vi "crossover detection.vi"(7 "reference line":dbl format="%#_13g", 8 "error in":errorcluster, 9 "Plot":dbl[][](array[numeric])) -> (0 "error out":errorcluster, 2 "crossovers":dbl[](array[numeric]))   [LabVIEW 2014]
panel:
  out "debouncing negative e":i32
  out "debouncing positive e.":i32
  out "n.e.c. validated":dbl[](array[numeric])
  out "p.e.c. validated":dbl[](array[numeric])
  out "positive edge\ncrossovers (x value)":dbl[](array[numeric])
  out "negative edge\ncorssovers (x value)":dbl[](array[numeric])
  # "For testing only"
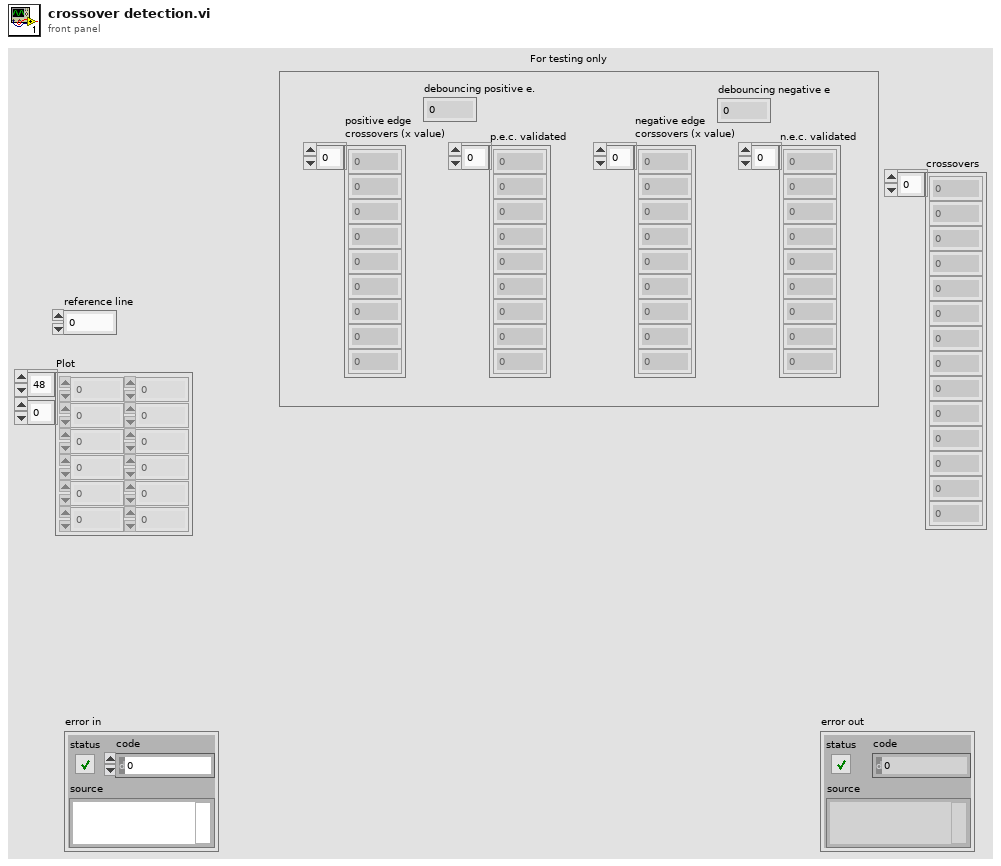
[diagram p1: front panel]
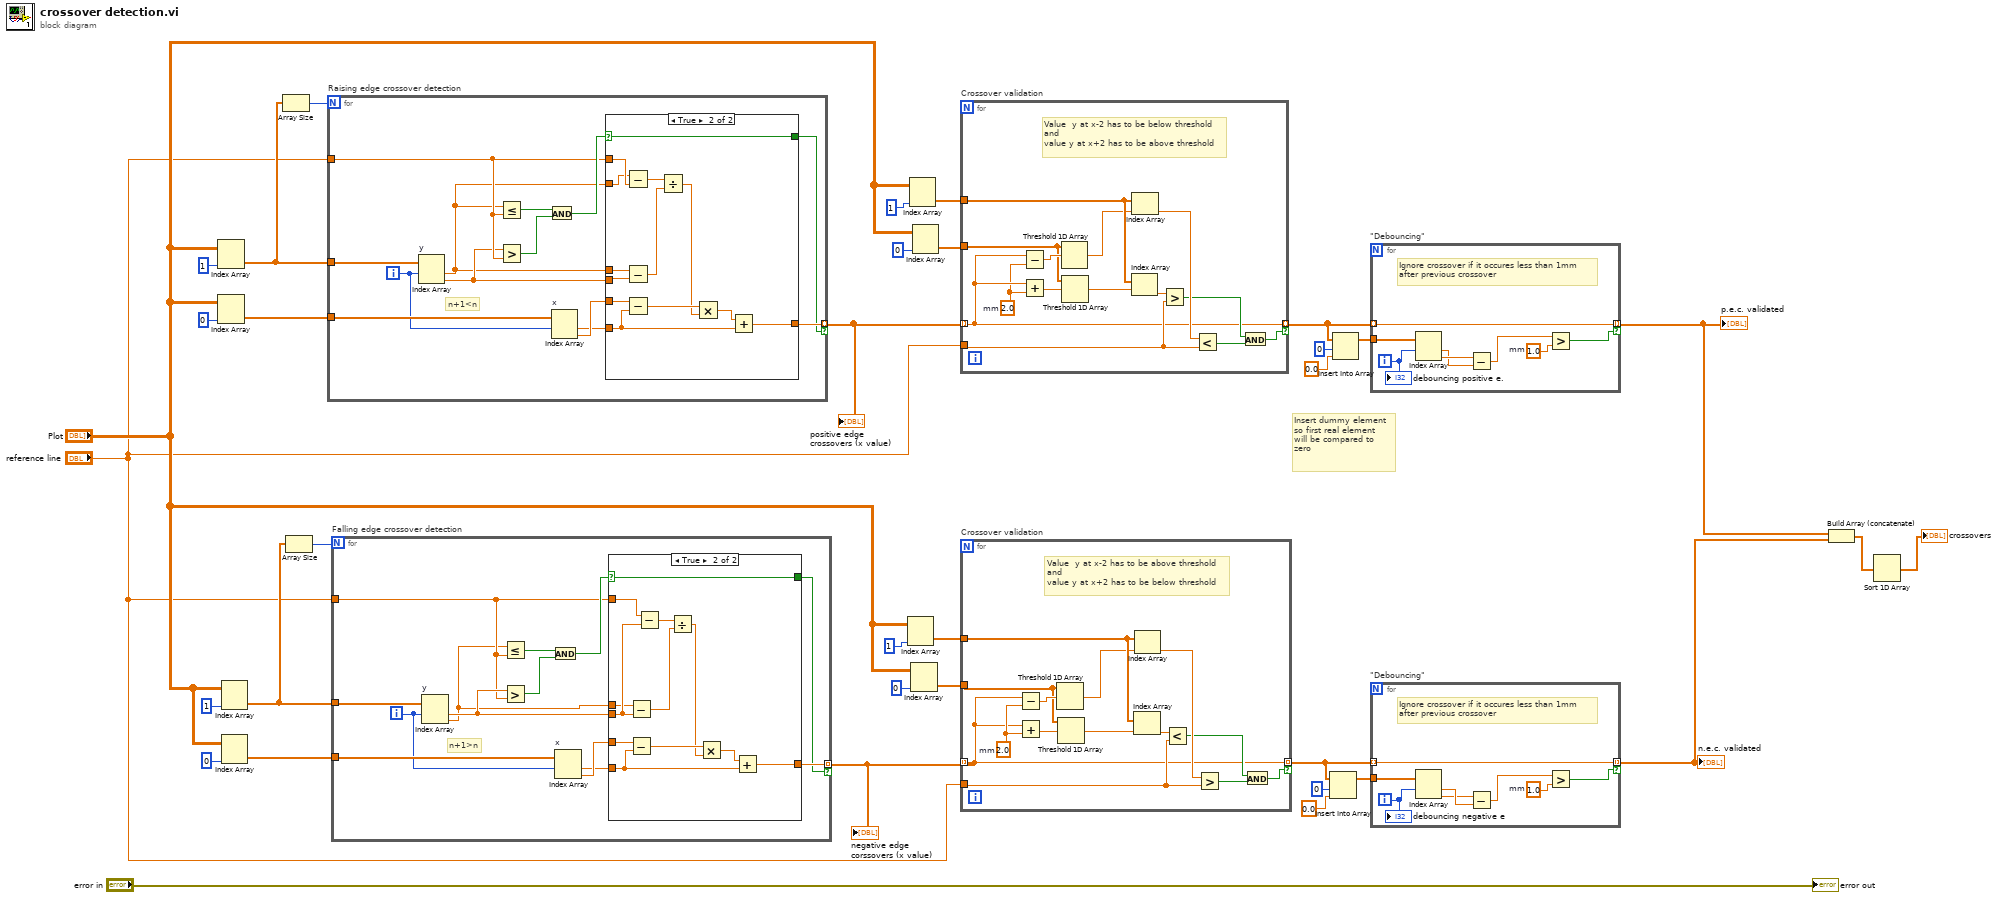
[diagram p0: block diagram]
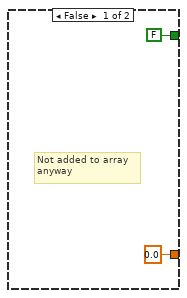
[diagram p2: hidden frame]
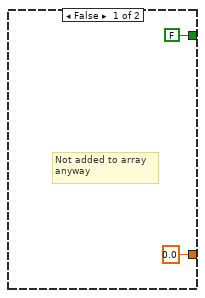
[diagram p3: hidden frame]
diagram:
  # "Insert dummy element so first real element will be compared to zero"
  n1 = Index Array(array="Plot", index (col)=1 ("index (row)")) -> (element=w32:dbl[])  [unwired: 1 in]
  n2 = Index Array(array="Plot", index (col)=0 ("index (row)")) -> (element=w31:dbl[])  [unwired: 1 in]
  n3 = Index Array(array="Plot", index (col)=1 ("index (row)")) -> (element=w27:dbl[])  [unwired: 1 in]
  n4 = Index Array(array="Plot", index (col)=0 ("index (row)")) -> (element=w26:dbl[])  [unwired: 1 in]
  n5 = Array Size(array=w32) -> (size(s)=w33:i32)
  n6 = Array Size(array=w27) -> (size(s)=w28:i32)
  n7 = for "Raising edge crossover detection" {
    N: w33 -> [_]
    tunnel: w32 -> [w48]
    tunnel: "reference line" -> [w42]
    tunnel: w31 -> [w44]
    tunnel: [w39] -> w19 mode=indexing if=w38
    i -> [w41]
    # "n+1<n"
    n8 = Index Array "y"(array=w48, index #1=w41) -> (element #1=w36:dbl, element #2=w40:dbl)  [unwired: 1 in]
    n9 = Less Or Equal?(x=w36, y=w42) -> (x <= y?=w47:bool)
    n10 = Greater?(x=w40, y=w42) -> (0:w46:bool)
    n11 = And(x=w47, y=w46) -> (x .and. y?=w45:bool)
    n12 = Index Array "x"(array=w44, index #1=w41) -> (element #1=w37:dbl, element #2=w43:dbl)  [unwired: 1 in]
    n13 = case shown="True" w45 {
      selector: w45 -> [_ w56]
      tunnel: w43 -> [_ w58]
      tunnel: w37 -> [_ w55]
      tunnel: w40 -> [_ w51]
      tunnel: w36 -> [_ w53]
      tunnel: w42 -> [_ w54]
      tunnel: [0.0 w57] -> w39
      tunnel: [FALSE w56] -> w38
      tunnel: w36 -> [_ w52]
      frame False {
        # "Not added to array \nanyway"
      }
      frame True {
        n14 = Subtract(x=w53, y=w54) -> (x-y=w62:dbl)
        n15 = Subtract(x=w52, y=w51) -> (x-y=w63:dbl)
        n16 = Subtract(x=w58, y=w55) -> (x-y=w61:dbl)
        n17 = Divide(x=w62, y=w63) -> (x/y=w60:dbl)
        n18 = Multiply(x=w61, y=w60) -> (x*y=w59:dbl)
        n19 = Add(x=w59, y=w55) -> (x+y=w57:dbl)
      }
    }
  }
  "positive edge\ncrossovers (x value)" <- w19
  n20 = for "Falling edge crossover detection" {
    N: w28 -> [_]
    tunnel: w27 -> [w76]
    tunnel: "reference line" -> [w65]
    tunnel: w26 -> [w72]
    tunnel: [w69] -> w12 mode=indexing if=w68
    i -> [w70]
    # "n+1>n"
    n21 = Index Array "y"(array=w76, index #1=w70) -> (element #1=w66:dbl, element #2=w64:dbl)  [unwired: 1 in]
    n22 = Less Or Equal?(x=w64, y=w65) -> (x <= y?=w75:bool)
    n23 = Greater?(x=w66, y=w65) -> (0:w74:bool)
    n24 = And(x=w75, y=w74) -> (x .and. y?=w73:bool)
    n25 = Index Array "x"(array=w72, index #1=w70) -> (element #1=w67:dbl, element #2=w71:dbl)  [unwired: 1 in]
    n26 = case shown="True" w73 {
      selector: w73 -> [_ w86]
      tunnel: w71 -> [_ w88]
      tunnel: w67 -> [_ w85]
      tunnel: w66 -> [_ w82]
      tunnel: [0.0 w87] -> w69
      tunnel: [FALSE w86] -> w68
      tunnel: w65 -> [_ w83]
      tunnel: w64 -> [_ w80]
      frame False {
        # "Not added to array \nanyway"
      }
      frame True {
        n27 = Subtract(x=w80, y=w82) -> (x-y=w81:dbl)
        n28 = Subtract(x=w88, y=w85) -> (x-y=w90:dbl)
        n29 = Subtract(x=w83, y=w82) -> (x-y=w84:dbl)
        n30 = Divide(x=w84, y=w81) -> (x/y=w79:dbl)
        n31 = Multiply(x=w90, y=w79) -> (x*y=w89:dbl)
        n32 = Add(x=w89, y=w85) -> (x+y=w87:dbl)
      }
    }
  }
  "negative edge\ncorssovers (x value)" <- w12
  n33 = Index Array(array="Plot", index (col)=1 ("index (row)")) -> (element=w14:dbl[])  [unwired: 1 in]
  n34 = Index Array(array="Plot", index (col)=1 ("index (row)")) -> (element=w18:dbl[])  [unwired: 1 in]
  n35 = Index Array(array="Plot", index (col)=0 ("index (row)")) -> (element=w13:dbl[])  [unwired: 1 in]
  n36 = Index Array(array="Plot", index (col)=0 ("index (row)")) -> (element=w20:dbl[])  [unwired: 1 in]
  n37 = for "Crossover validation" {
    tunnel: w19 -> [w95] mode=indexing
    tunnel: w20 -> [w93]
    tunnel: w18 -> [w103]
    tunnel: "reference line" -> [w101]
    tunnel: [w95] -> w8 mode=indexing if=w98
    w94 = 2.0  # mm
    # "Value  y at x-2 has to be below threshold\nand\nvalue y at x+2 has to be above threshold"
    n38 = Subtract(x=w95, y=w94) -> (x-y=w97:dbl)
    n39 = Add(x=w95, y=w94) -> (x+y=w92:dbl)
    n40 = Threshold 1D Array(2:w97, 3:w93) -> (0:w96:dbl)  [unwired: 1 in]
    n41 = Threshold 1D Array(2:w92, 3:w93) -> (0:w91:dbl)  [unwired: 1 in]
    n42 = Index Array(array=w103, index=w91) -> (element=w102:dbl)
    n43 = Index Array(array=w103, index=w96) -> (element=w104:dbl)
    n44 = Greater?(x=w102, y=w101) -> (0:w99:bool)
    n45 = Less?(x=w104, y=w101) -> (x < y?=w100:bool)
    n46 = And(x=w99, y=w100) -> (x .and. y?=w98:bool)
  }
  n47 = for "Crossover validation" {
    tunnel: w12 -> [w105] mode=indexing
    tunnel: w13 -> [w108]
    tunnel: w14 -> [w117]
    tunnel: "reference line" -> [w115]
    tunnel: [w105] -> w1 mode=indexing if=w112
    w110 = 2.0  # mm
    # "Value  y at x-2 has to be above threshold\nand\nvalue y at x+2 has to be below threshold"
    n48 = Subtract(x=w105, y=w110) -> (x-y=w111:dbl)
    n49 = Add(x=w105, y=w110) -> (x+y=w109:dbl)
    n50 = Threshold 1D Array(2:w111, 3:w108) -> (0:w107:dbl)  [unwired: 1 in]
    n51 = Threshold 1D Array(2:w109, 3:w108) -> (0:w106:dbl)  [unwired: 1 in]
    n52 = Index Array(array=w117, index=w106) -> (element=w116:dbl)
    n53 = Index Array(array=w117, index=w107) -> (element=w118:dbl)
    n54 = Less?(x=w116, y=w115) -> (x < y?=w113:bool)
    n55 = Greater?(x=w118, y=w115) -> (0:w114:bool)
    n56 = And(x=w113, y=w114) -> (x .and. y?=w112:bool)
  }
  n57 = Insert Into Array(array=w1, index=0, new element=0.0 ("new element/subarray")) -> (w2:dbl[])
  n58 = Insert Into Array(array=w8, index=0, new element=0.0 ("new element/subarray")) -> (w7:dbl[])
  n59 = for "\"Debouncing\"" {
    tunnel: w7 -> [w126]
    tunnel: w8 -> [w122] mode=indexing
    tunnel: [w122] -> w10 mode=indexing if=w121
    i -> [w125]
    w123 = 1.0  # mm
    # "Ignore crossover if it occures less than 1mm\nafter previous crossover"
    n60 = Index Array(array=w126, index #1=w125) -> (element #1=w119:dbl, element #2=w120:dbl)  [unwired: 1 in]
    n61 = Subtract(x=w120, y=w119) -> (x-y=w124:dbl)
    n62 = Greater?(x=w124, y=w123) -> (0:w121:bool)
    "debouncing positive e." <- w125
  }
  "p.e.c. validated" <- w10
  n63 = for "\"Debouncing\"" {
    tunnel: w2 -> [w134]
    tunnel: w1 -> [w130] mode=indexing
    tunnel: [w130] -> w9 mode=indexing if=w129
    i -> [w133]
    w131 = 1.0  # mm
    # "Ignore crossover if it occures less than 1mm\nafter previous crossover"
    n64 = Index Array(array=w134, index #1=w133) -> (element #1=w128:dbl, element #2=w127:dbl)  [unwired: 1 in]
    n65 = Subtract(x=w127, y=w128) -> (x-y=w132:dbl)
    n66 = Greater?(x=w132, y=w131) -> (0:w129:bool)
    "debouncing negative e" <- w133
  }
  "n.e.c. validated" <- w9
  n67 = Build Array (concatenate)(w10, w9) -> (w23:dbl[])
  n68 = Sort 1D Array(array=w23) -> (sorted array=→"crossovers":dbl[])
  "error out" <- "error in"
